vi "Vacuum and Terminal Monitor.vi"() -> ()   [LabVIEW 2016, in "Top Level.lvlib"]
doc: "This VI is part of the Top Level library of VIs that are opened upon startup. Vacuum pressures are read via serial connections between the vacuum gauge controller and the nearest cRIO. At the cRIO, a Real-Time VI puts the pressures into shared variables which are displayed here."
uses:
  Top Level.lvlib
panel:
  in  "Tab Control":enum32{"Readbacks", "Errors"}(tab)
  out "LE Waist":string
  out "Tank Entrance":string
  out "Tank Exit":string
  out "Analyzer Image":string
  out "HE Waist/Analyzer Object":string
  out "Transmission":string
  out "R30 Switch Image":string
  out "R30 Detector":string
  out "R30 ESA":string
  in  "stop":bool
  out "date/time string":string
  out "Injector A Image":string
  out "Injector A Object":string
  out "Terminal Voltage":dbl format="%#_4g"
  out "R45 EXB":string
  out "R45 Switch Image":string
  out "R45 Waist":string
  out "SCA bellows":string
  out "SCA source":string
  out "SV read error":errorcluster
  out "Terminal read error":errorcluster
  out "Cryo readback error":errorcluster
  out "R45 switch Cryo pump":T1
  out "R30 ESA Cryo pump":T1
  out "Inj image Cryo pump":T2
  # "VACUUM  PRESSURES"
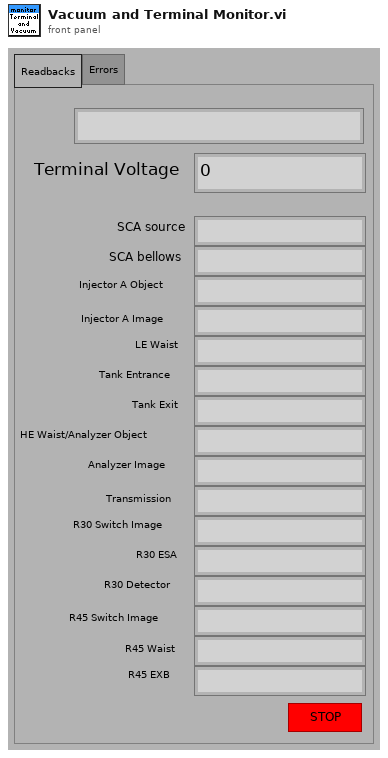
[diagram p1: front panel]
types:
  T1 = cluster{"First Stage":dbl, "Second stage":dbl, "Hours since last regen":dbl, "Pump ON":bool, "Time on":dbl}
  T2 = cluster{"First Stage":dbl, "Second stage":dbl, "Last regen":dbl, "Pump ON":bool, "Time on":dbl}
  T3 = cluster{"Ion gauge 1":string, "Convectron  Gauge 1 ":string, "Ion Gauge 2":string, "Convectrom Gauge 2":string}
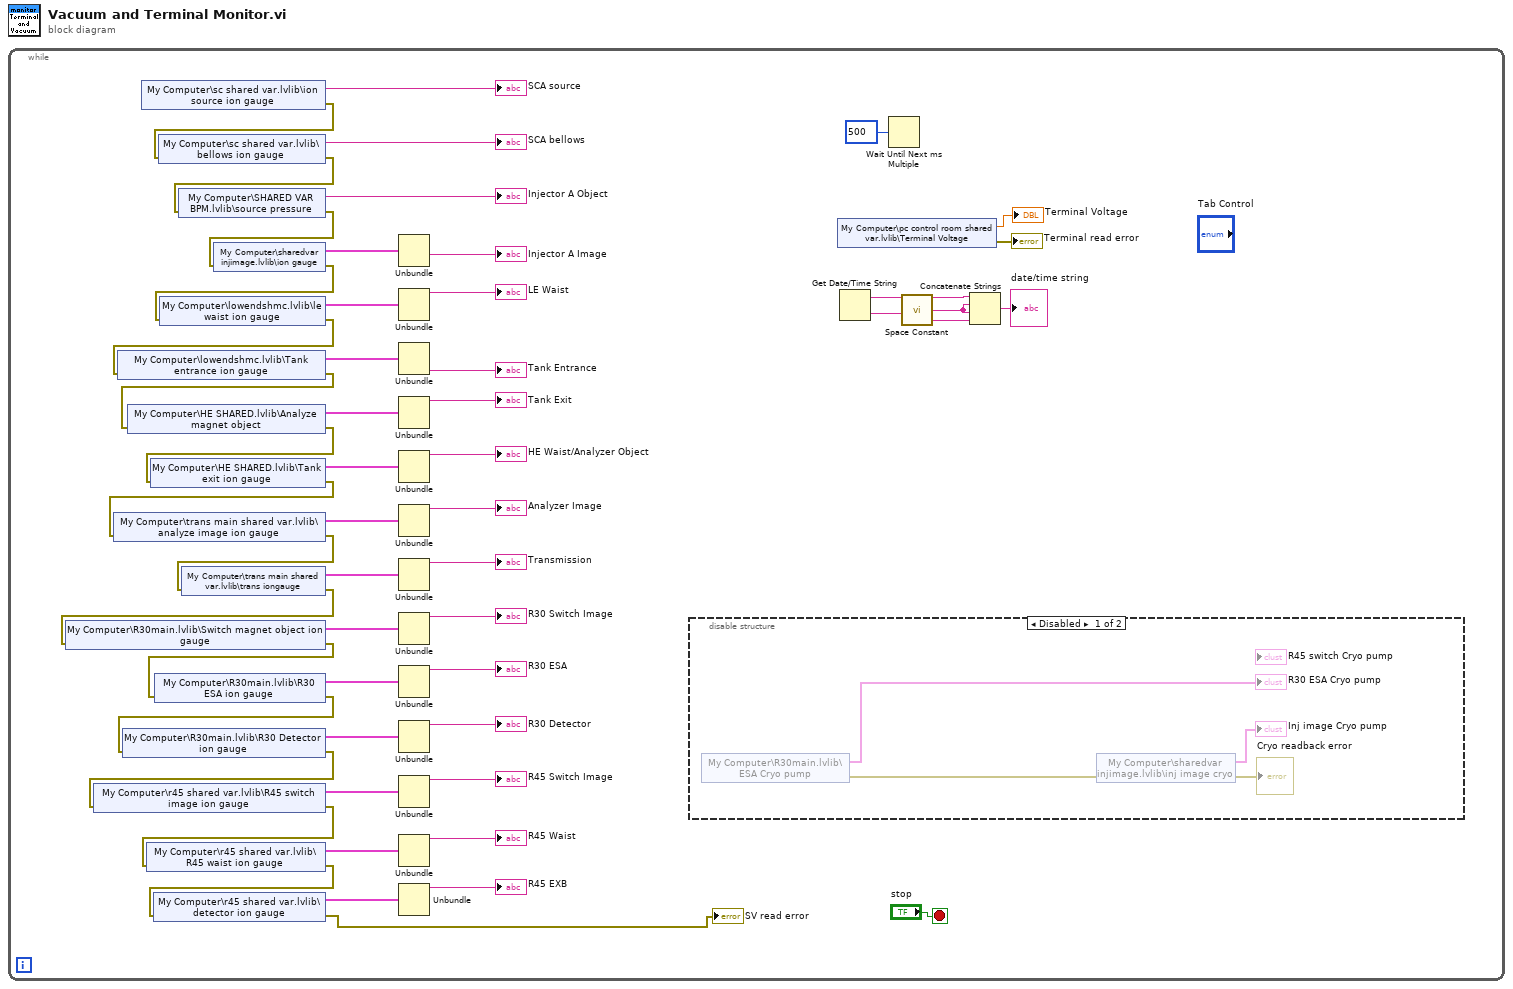
[diagram p0: block diagram]
diagram:
  n1 = while {
    stop <- "stop" stop-if-true
    n2 = shared-variable "My Computer\\sc shared var.lvlib\\ion source ion gauge"() -> (→"SCA source":string, error out=w16:errorcluster)  [unwired: 1 in]
    n3 = shared-variable "My Computer\\sc shared var.lvlib\\bellows ion gauge"(error in=w16) -> (→"SCA bellows":string, error out=w15:errorcluster)
    n4 = shared-variable "My Computer\\SHARED VAR BPM.lvlib\\source pressure"(error in=w15) -> (→"Injector A Object":string, error out=w14:errorcluster)
    n5 = shared-variable "My Computer\\sharedvar injimage.lvlib\\ion gauge"(error in=w14) -> (w47:cluster{string, string, string, string}, error out=w13:errorcluster)
    n6 = shared-variable "My Computer\\lowendshmc.lvlib\\le waist ion gauge"(error in=w13) -> (w51:cluster{string, string, string, string}, error out=w12:errorcluster)
    n7 = shared-variable "My Computer\\lowendshmc.lvlib\\Tank entrance ion gauge"(error in=w12) -> (w50:cluster{string, string, string, string}, error out=w11:errorcluster)
    n8 = shared-variable "My Computer\\HE SHARED.lvlib\\Analyze magnet object"(error in=w11) -> (w49:cluster{string, string, string, string}, error out=w10:errorcluster)
    n9 = shared-variable "My Computer\\HE SHARED.lvlib\\Tank exit ion gauge"(error in=w10) -> (w48:cluster{string, string, string, string}, error out=w9:errorcluster)
    n10 = shared-variable "My Computer\\trans main shared var.lvlib\\analyze image ion gauge"(error in=w9) -> (w41:T3, error out=w8:errorcluster)
    n11 = shared-variable "My Computer\\trans main shared var.lvlib\\trans iongauge"(error in=w8) -> (w40:T3, error out=w7:errorcluster)
    n12 = shared-variable "My Computer\\R30main.lvlib\\Switch magnet object ion gauge"(error in=w7) -> (w39:cluster{string, string, string, string}, error out=w6:errorcluster)
    n13 = shared-variable "My Computer\\R30main.lvlib\\R30 ESA ion gauge"(error in=w6) -> (w37:cluster{string, string, string, string}, error out=w5:errorcluster)
    n14 = shared-variable "My Computer\\R30main.lvlib\\R30 Detector ion gauge"(error in=w5) -> (w38:cluster{string, string, string, string}, error out=w4:errorcluster)
    n15 = shared-variable "My Computer\\r45 shared var.lvlib\\R45 switch image ion gauge"(error in=w4) -> (w34:T3, error out=w3:errorcluster)
    n16 = shared-variable "My Computer\\r45 shared var.lvlib\\R45 waist ion gauge"(error in=w3) -> (w33:T3, error out=w2:errorcluster)
    n17 = shared-variable "My Computer\\r45 shared var.lvlib\\detector ion gauge"(error in=w2) -> (w35:T3, error out=→"SV read error":errorcluster)
    n18 = Unbundle(w47) -> (→"Injector A Image":string)  [unwired: 3 out]
    n19 = Unbundle(w51) -> (→"LE Waist":string)  [unwired: 3 out]
    n20 = Unbundle(w50) -> (→"Tank Entrance":string)  [unwired: 3 out]
    n21 = Unbundle(w49) -> (→"Tank Exit":string)  [unwired: 3 out]
    n22 = Unbundle(w48) -> (→"HE Waist/Analyzer Object":string)  [unwired: 3 out]
    n23 = Unbundle(w41) -> ("Ion gauge 1"=→"Analyzer Image":string)  [unwired: 3 out]
    n24 = Unbundle(w40) -> ("Ion gauge 1"=→"Transmission":string)  [unwired: 3 out]
    n25 = Unbundle(w39) -> (→"R30 Switch Image":string)  [unwired: 3 out]
    n26 = Unbundle(w37) -> (→"R30 ESA":string)  [unwired: 3 out]
    n27 = Unbundle(w38) -> (→"R30 Detector":string)  [unwired: 3 out]
    n28 = Unbundle(w34) -> ("Ion gauge 1"=→"R45 Switch Image":string)  [unwired: 3 out]
    n29 = Unbundle(w33) -> ("Ion gauge 1"=→"R45 Waist":string)  [unwired: 3 out]
    n30 = Unbundle(w35) -> ("Ion gauge 1"=→"R45 EXB":string)  [unwired: 3 out]
    n31 = disable-structure shown="Disabled" {
      frame Disabled {
        n32 = shared-variable "My Computer\\R30main.lvlib\\ESA Cryo pump"() -> (→"R30 ESA Cryo pump":T1, error out=w54:errorcluster)  [unwired: 1 in]
        n33 = shared-variable "My Computer\\sharedvar injimage.lvlib\\inj image cryo"(error in=w54) -> (→"Inj image Cryo pump":T1, error out=→"Cryo readback error":errorcluster)
      }
      frame Enabled {
      }
    }
    n34 = shared-variable "My Computer\\pc control room shared var.lvlib\\Terminal Voltage"() -> (→"Terminal Voltage":dbl, error out=→"Terminal read error":errorcluster)  [unwired: 1 in]
    n35 = Get Date/Time String() -> (date string=w45:string, time string=w42:string)  [unwired: 3 in]
    n36 = Wait Until Next ms Multiple(millisecond multiple=u32 500) -> ()  [unwired: 1 out]
    n37 = call <vilib>:"Space Constant.vi"() -> ("String"=w43:string)
    n38 = Concatenate Strings(w45, w43, w43, w42) -> (→"date/time string":string)
  }
